vi "Get PWMin references.vi"(8 "error in (no error)":errorcluster, 10 "PWM in data":T1[](array[typedef]), 11 "Bitfile ref in":refnum<k20>) -> (0 "error out":errorcluster, 2 "PWM in data(RT)":T2[](array[typedef]))   [LabVIEW 2013, in "PWM Engine.lvlib"]
uses:
  PWM Engine.lvlib
  Shared/Types/PWM in info(RT).ctl
  Shared/Types/PWM in info.ctl
  <vilib>/NI/LVFPGA Adv Session Resources/OpenByNameSubVI.vi
  <vilib>/rvi/interface/common/dynamic/niFpgaEscapeDelimiterAndNull.vi
  <vilib>/Utility/error.llb/Error Cluster From Error Code.vi
  <vilib>/rvi/interface/common/niFpgaWaitOnOcc.vi
  <vilib>/rvi/errors/niLvFpgaAdjustHostInterfaceError.vi
  <vilib>/FPGAPlugInAG/Dynamic/niLvFpga_Close_Dynamic.vi
  <vilib>/NI/LVFPGA Adv Session Resources/OpenByName.xnode
  <vilib>/rvi/interface/nirviReadWriteControl/nirviReadWriteControl.xnode
  <vilib>/rvi/interface/nirviCloseFPGA/nirviCloseFPGA.xnode
  <vilib>/NI/LVFPGA Adv Session Resources/LVFPGAAdvSessionResources.lvlib
  NiFpgaLv.dll
  <vilib>/rvi/interface/Simulation/niFpgaSimulationCallBeginRW.vi
  Shared/PWM Shared.lvlib
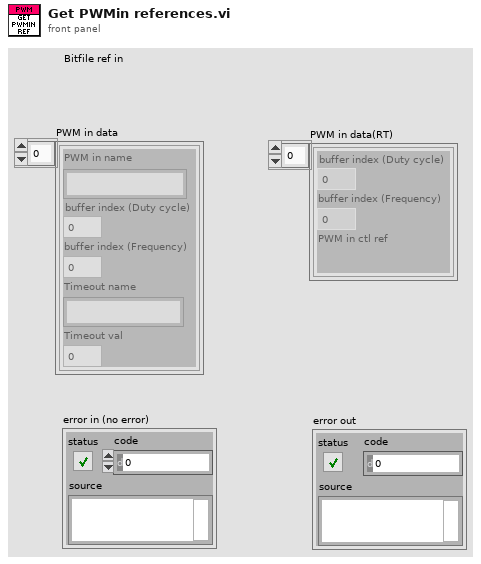
[diagram p1: front panel]
types:
  T1 = typedef "PWM Shared.lvlib/PWM in info.ctl" = cluster{"PWM in name":string, "buffer index (Duty cycle)":i32, "buffer index (Frequency)":i32, "Timeout name":string, "Timeout val":dbl}
  T2 = typedef "PWM Shared.lvlib/PWM in info(RT).ctl" = cluster{"buffer index (Duty cycle)":i32, "buffer index (Frequency)":i32, "PWM in ctl ref":refnum<k20>}
  T3 = cluster{"Name":string, "Depth":u32, "Write? (Deprecated:Use Implementation)":bool, "Physical Channel":u32, "Base Address":u32, "Data Width":u32, "Data Type":enum32{"Boolean", "I8", "I16", "I32", "I64", "U8", "U16", "U32", "U64", "FXP", "CustomControl", "SGL"}, "FXP Properties":variant, "Write Window Address":u32, "Implementation":enum16{"niFpgaTargetToHost", "niFpgaHostToTarget", "niFpgaPeerToPeerWriter", "niFpgaPeerToPeerReader", "niCoreTargetToHost", "niCoreHostToTarget"}, "Control Set":u32}[]
  T4 = cluster{"Name":string, "type":variant, "indicator?":bool}[]
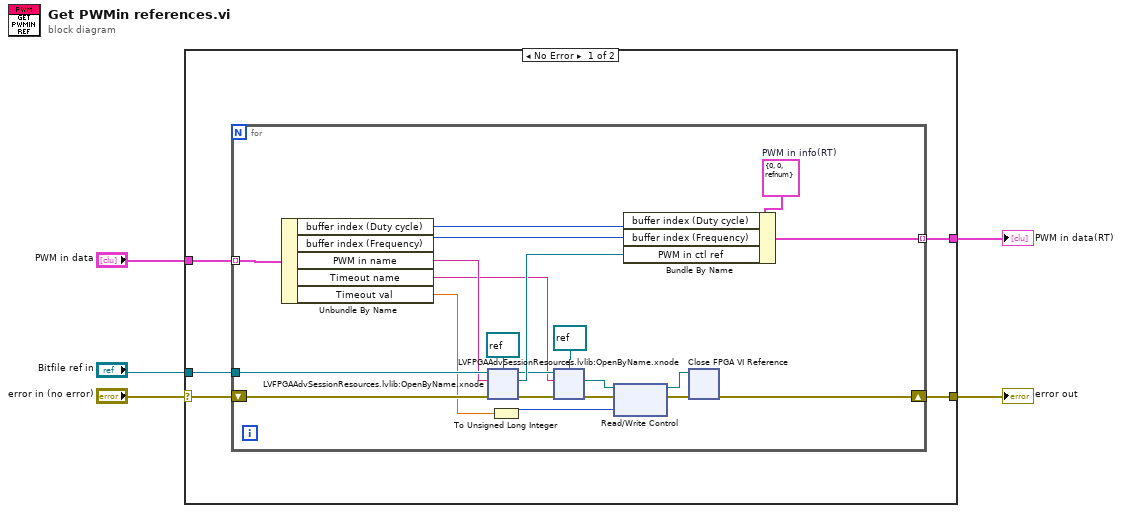
[diagram p0: block diagram]
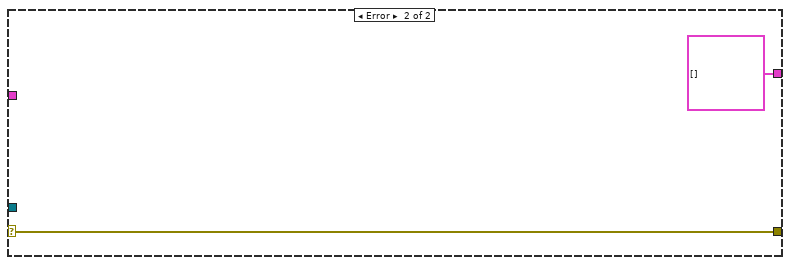
[diagram p2: hidden frame]
diagram:
  n1 = case shown="No Error" "error in (no error)" {
    selector: "error in (no error)" -> [w6 w59]
    tunnel: [w10 T2[] []] -> w5
    tunnel: "Bitfile ref in" -> [w9 _]
    tunnel: [w8 w59] -> w3
    tunnel: "PWM in data" -> [w7 _]
    frame No Error {
      n2 = for {
        shift-right: [w12] -> w8
        shift-left: w6 -> [w30]
        tunnel: w7 -> [w19] mode=indexing
        tunnel: [w20] -> w10 mode=indexing
        tunnel: w9 -> [w31]
        w18 = T2 {"buffer index (Duty cycle)"=0, "buffer index (Frequency)"=0, "PWM in ctl ref"=refnum}  # PWM in info(RT)
        n3 = Unbundle By Name(w19) -> ("buffer index (Duty cycle)"=w17:i32, "buffer index (Frequency)"=w16:i32, "PWM in name"=w29:string, "Timeout name"=w21:string, "Timeout val"=w22:dbl)
        n4 = xnode "LVFPGAAdvSessionResources.lvlib:OpenByName.xnode"("FPGA VI Reference in"=w31, "Resource name in"=w29, "Single resource reference type in"=refnum<k20> refnum ("FPGA Interface"), "Error in"=w30) -> ("Single resource reference out"=w28:refnum<k20>, "Error out"=w27:errorcluster, "FPGA VI Reference out"=w26:refnum<k20>)
        n5 = To Unsigned Long Integer(number=w22) -> (unsigned 32bit integer=w15:u32)
        n6 = xnode "LVFPGAAdvSessionResources.lvlib:OpenByName.xnode"("FPGA VI Reference in"=w26, "Resource name in"=w21, "Single resource reference type in"=refnum<k20> refnum ("FPGA Interface"), "Error in"=w27) -> ("Single resource reference out"=w23:refnum<k20>, "Error out"=w25:errorcluster)  [unwired: 1 out]
        n7 = xnode "Read/Write Control"("FPGA VI Reference In"=w23, "error in"=w25, "Value"=w15) -> ("FPGA VI Reference Out"=w11:refnum<k20>, "error out"=w13:errorcluster)
        n8 = Bundle By Name(cluster=w18, "buffer index (Duty cycle)"=w17, "buffer index (Frequency)"=w16, "PWM in ctl ref"=w28) -> (w20:T2)
        n9 = xnode "Close FPGA VI Reference"("FPGA VI Reference In"=w11, "error in"=w13) -> ("error out"=w12:errorcluster)
      }
    }
    frame Error {
    }
  }
  "PWM in data(RT)" <- w5
  "error out" <- w3
